vi "create ref image (subVI).vi"(10 "Array in":u16[][][](array[numeric]), 11 "config in":T1) -> (2 "ref image":u16[][](array[numeric]), 3 "Waveform Graph":u32[](graph))   [LabVIEW 2024]
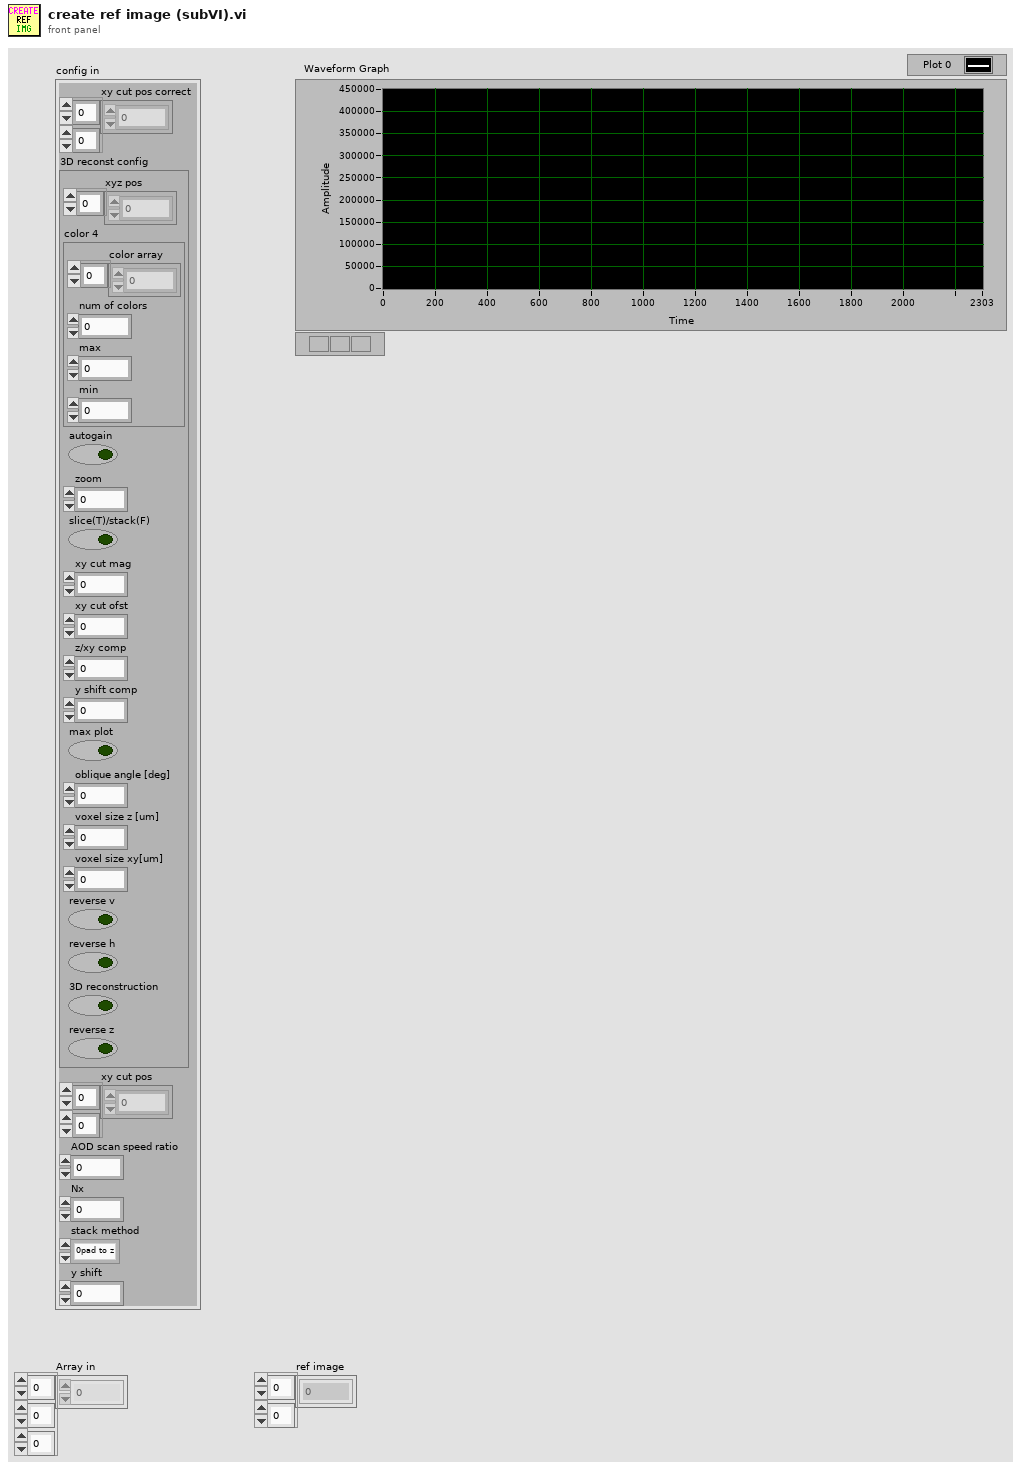
[diagram p1: front panel]
types:
  T1 = cluster{"xy cut pos correct":dbl[][], "3D reconst config":cluster{"xyz pos":u16[], "color 4":cluster{"color array":u32[], "num of colors":i32, "max":dbl, "min":dbl}, "autogain":bool, "zoom":dbl, "slice(T)/stack(F)":bool, "xy cut mag":dbl, "xy cut ofst":dbl, "z/xy comp":dbl, "y shift comp":dbl, "max plot":bool, "oblique angle [deg]":dbl, "voxel size z [um]":dbl, "voxel size xy[um]":dbl, "reverse v":bool, "reverse h":bool, "3D reconstruction":bool, "reverse z":bool}, "xy cut pos":dbl[][], "AOD scan speed ratio":dbl, "Nx":dbl, "stack method":enum16{"0pad to z", "0pad to x", "0pad to x and rot"}, "y shift":i32}
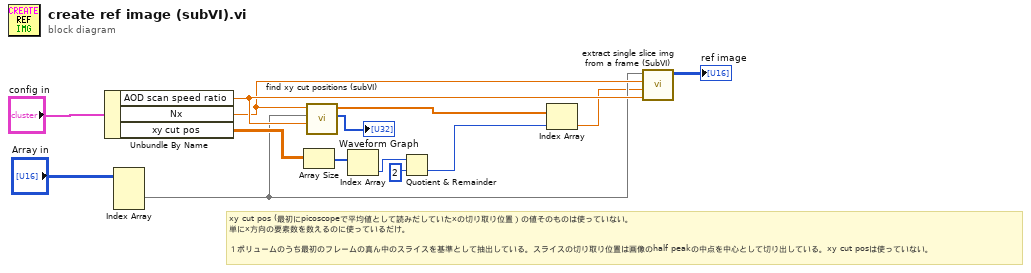
[diagram p0: block diagram]
diagram:
  # "xy cut pos (最初にpicoscopeで平均値として読みだしていたxの切り取り位置）の値そのものは使っていない。\n単にx方向の要素数を数えるのに使っているだけ。\n\n１ボリュームのうち最初のフレームの真ん中のスライスを基準として抽出している。スライスの切り取り位置は画像のhalf peakの中点を中心として切り出している。xy cut posは使っていない。"
  n1 = Unbundle By Name("config in") -> ("AOD scan speed ratio"=w13:dbl, "Nx"=w12:dbl, "xy cut pos"=w14:dbl[][])
  n2 = Index Array(array="Array in") -> (element=w5:u16[][])  [unwired: 3 in]
  n3 = Array Size(array=w14) -> (size(s)=w7:i32[])
  n4 = call "find xy cut positions (subVI).vi"("r"=w13, "input frame"=w5, "Nx"=w12) -> ("projection profiles"=→"Waveform Graph":u32[], "xy cut positions"=w2:dbl[])  [unwired: 7 in]
  n5 = Index Array(array=w7) -> (element=w8:i32)  [unwired: 1 in]
  n6 = Quotient & Remainder(x=w8, y=2) -> (floor(x/y)=w10:i32)  [unwired: 1 out]
  n7 = Index Array(array=w2, index=w10) -> (element=w3:dbl)
  n8 = call "extract single slice img from a frame (SubVI).vi"("AOD scan speed ratio"=w13, "init pos"=w3, "Nx"=w12, "image in"=w5) -> ("Array"=→"ref image":u16[][])  [unwired: 7 in]
